vi "Waveform Replication (Simulated).vi"() -> ()   [LabVIEW 2019]
doc: "This example demonstrates how to apply an LMS adaptive filter to road simulation applications. Road simulation is one of waveform replication applicaitons. Road simulation is to replicate a vibration waveform through a shaker. This example simulates a shaker with an FIR filter, uses an LMS adptive filter to build the inverse model of the shaker, and uses this inverse model to regulate the driving signal for the shaker so that the shaker produces expected waveforms exactly.\n\nRun the VI, and observe the inverse model of the shaker and the comparision between the actual and expected shaker output.\n\nIf <b>Closed Loop</b> is FALSE, this example applies the original waveform to the shaker. Notice that the actual shaker output is much different from the expected shaker output.\n\nIf <b>Closed Loop</b> is TRUE, this example regulates the original waveform with the inverse model of the shaker and then applies the waveform to the shaker. Notice that the actual shaker output is much closer to the expected shaker output."
uses:
  <vilib>/addons/Adaptive Filters/Create/AFT Create FIR LMS (Real).vi
  <vilib>/Analysis/3filter.llb/FIR Filter (DBL).vi
  <vilib>/addons/Adaptive Filters/Processing/AFT Filter Signal and Update Coefficients (Real, Array).vi
  <vilib>/addons/Adaptive Filters/Analysis/AFT Get Coefficients (FIR, Real).vi
  <vilib>/addons/Adaptive Filters/NI_AdaptiveFilter.lvlib
  <vilib>/Analysis/NI_AALBase.lvlib
panel:
  in  "Tab Control":enum32{"Background", "Road Simulation Control"}(tab)
  in  "Closed Loop":bool
  out "H(z) - Inverse Model of the Shaker":dbl[](graph)
  out "Signals":dbl[][](graph)
  in  "Filter Length":i32=500 min=2
  in  "Step Size":dbl=0.01 min=0.0 step=0.01
  in  "Delay":i32=300 min=0
  in  "Stop":bool
  # "Waveform replication is to let mechanical or electrical devices replicate an expected waveform exactly. Waveform replication is one of adaptive inverse control applications. Refer to the Adaptive Inverse Control topic in the LabVIEW Help for more information about the background of adaptive inverse control. Select Help>>Show Context Help and move the cursor over the VI icon of this example for more information."
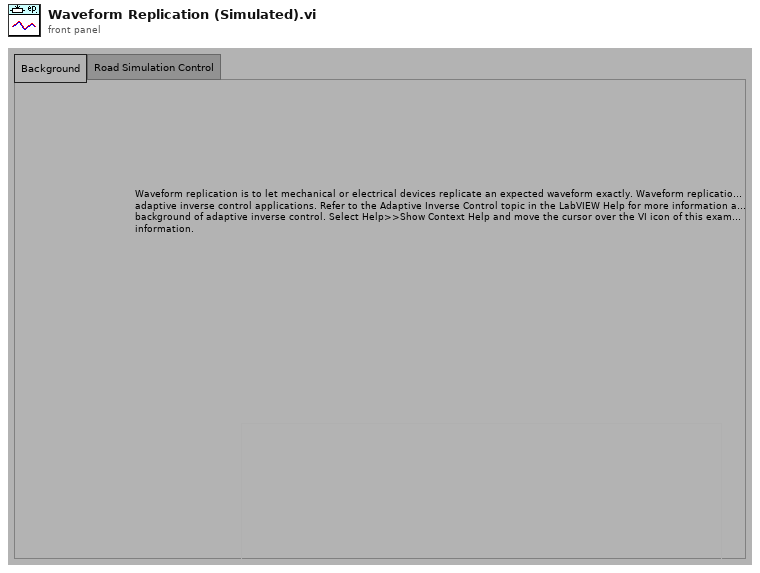
[diagram p1: front panel]
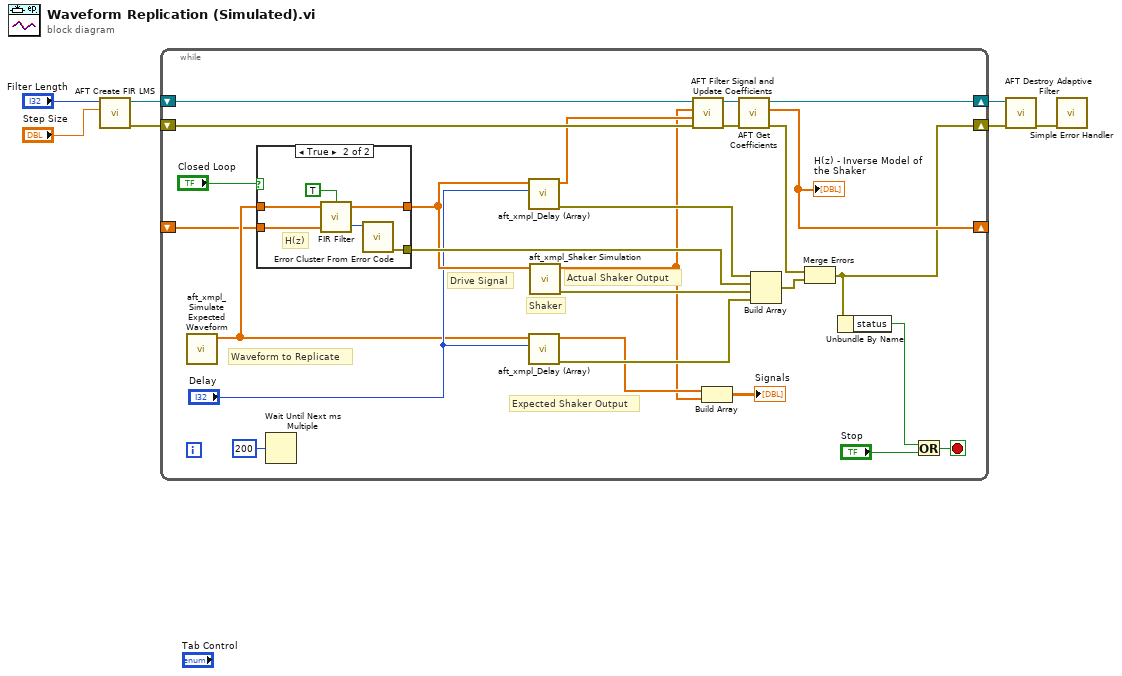
[diagram p0: block diagram]
diagram:
  n1 = call-poly <vilib>:"AFT Create FIR LMS.vi"("step size"="Step Size", "filter length"="Filter Length") -> ("error out"=w3:errorcluster, "adaptive filter out"=w6:refnum<k20>)  [unwired: 2 in, 6 out]
  n2 = while {
    shift-right: [w16] -> _
    shift-left: _ -> [w15]
    shift-right: [w10] -> w2
    shift-left: w3 -> [w25]
    shift-right: [w27] -> w4
    shift-left: w6 -> [w28]
    stop <- w9 stop-if-true
    # "Shaker"
    # "Drive Signal"
    # "Expected Shaker Output"
    # "Actual Shaker Output"
    # "Waveform to Replicate"
    n3 = call "aft_xmpl_Simulate Expected Waveform.vi"() -> ("Expected Waveform"=w18:dbl[])  [unwired: 11 out]
    n4 = case shown="True" "Closed Loop" {
      tunnel: [w34 w40] -> w29
      tunnel: w18 -> [w34 w39]
      tunnel: w15 -> [_ w37]
      tunnel: [_ w35] -> w32
      frame False {
      }
      frame True {
        # "H(z)"
        n5 = call-poly <vilib>:"FIR Filter.vi"("init/cont (init:F)"=TRUE, "FIR Coefficients"=w37, "X"=w39) -> ("error"=w36:i32, "Filtered X"=w40:dbl[])  [unwired: 1 out]
        n6 = call <vilib>:"Error Cluster From Error Code.vi"("error code (0)"=w36) -> ("error out"=w35:errorcluster)  [unwired: 2 in, 6 out]
      }
    }
    n7 = Wait Until Next ms Multiple(millisecond multiple=u32 200) -> ()  [unwired: 1 out]
    n8 = call "aft_xmpl_Delay (Array).vi"("delay"="Delay", "X"=w29) -> ("error out"=w33:errorcluster, "Delayed X"=w14:dbl[])  [unwired: 1 in, 7 out]
    n9 = call "aft_xmpl_Delay (Array).vi"("delay"="Delay", "X"=w18) -> ("error out"=w30:errorcluster, "Delayed X"=w19:dbl[])  [unwired: 1 in, 7 out]
    n10 = call "aft_xmpl_Shaker Simulation.vi"("drive signal"=w29) -> ("error out"=w31:errorcluster, "shaker output"=w13:dbl[])  [unwired: 1 in, 8 out]
    n11 = call-poly <vilib>:"AFT Filter Signal and Update Coefficients.vi"("error in (no error)"=w25, "d(n)"=w14, "x(n)"=w13, "adaptive filter in"=w28) -> ("error out"=w24:errorcluster, "adaptive filter out"=w26:refnum<k20>)  [unwired: 2 in, 4 out]
    n12 = Build Array(w19, w13) -> (→"Signals":dbl[][])
    n13 = call-poly <vilib>:"AFT Get Coefficients.vi"("error in (no error)"=w24, "adaptive filter in"=w26) -> ("error out"=w12:errorcluster, "coefficients"=w16:dbl[], "adaptive filter out"=w27:refnum<k20>)  [unwired: 7 out]
    "H(z) - Inverse Model of the Shaker" <- w16
    n14 = Build Array(w33, w32, w31, w30) -> (w11:errorcluster[])
    n15 = Merge Errors(w12, w11) -> (w10:errorcluster)
    n16 = Unbundle By Name(w10) -> ("status"=w8:bool)
    n17 = Or(x=w8, y="Stop") -> (x .or. y?=w9:bool)
  }
  n18 = call <vilib>:"AFT Destroy Adaptive Filter.vi"("error in (no error)"=w2, "adaptive filter in"=w4) -> ("error out"=w1:errorcluster)  [unwired: 9 out]
  n19 = call <vilib>:"Simple Error Handler.vi"("error in (no error)"=w1) -> ()  [unwired: 1 in, 8 out]
